vi "CMN_testmessage.vi"(8 "error in (no error)":errorcluster, 11 "message  in":string) -> (0 "error out":errorcluster, 1 "TIMEOUT":bool, 2 "ERROR":bool, 3 "message out":string)   [LabVIEW 2016]
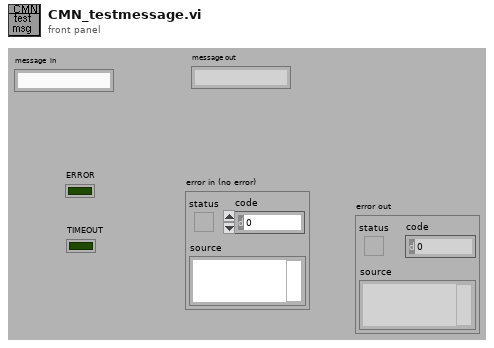
[diagram p1: front panel]
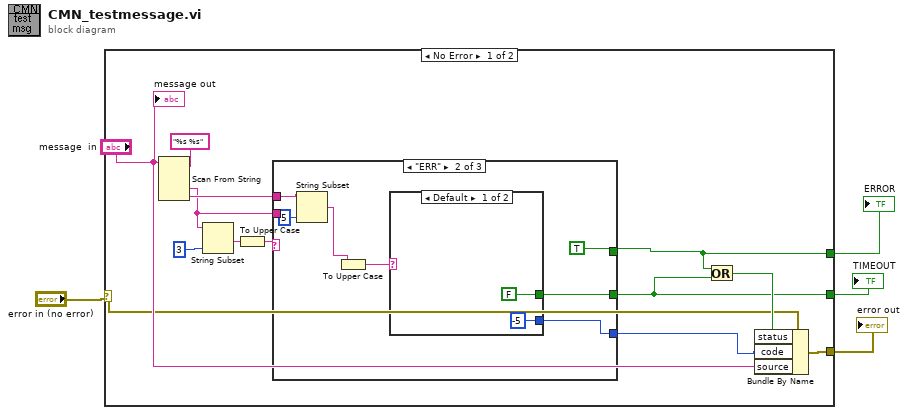
[diagram p0: block diagram]
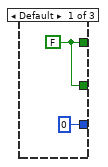
[diagram p2: hidden frame]
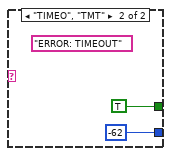
[diagram p3: hidden frame]
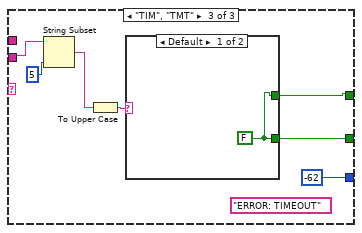
[diagram p4: hidden frame]
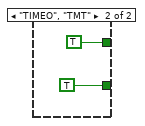
[diagram p5: hidden frame]
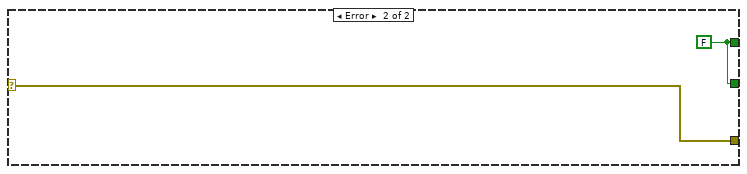
[diagram p6: hidden frame]
diagram:
  n1 = case shown="No Error" "error in (no error)" {
    selector: "error in (no error)" -> [w7 w41]
    tunnel: [w10 w41] -> w4
    tunnel: [w6 w42] -> w2
    tunnel: [w5 w42] -> w1
    frame No Error {
      n2 = Scan From String(format string="%s %s", input string="message  in") -> (output 1=w12:string, output 2=w13:string)  [unwired: 2 in, 5 out]
      n3 = String Subset(string=w12, length (rest)=3 ("length (rest)")) -> (substring=w15:string)  [unwired: 1 out]
      n4 = To Upper Case(1:w15) -> (0:w14:string)
      n5 = case shown="\"ERR\"" w14 {
        tunnel: [w19 TRUE w32] -> w5
        tunnel: w13 -> [_ w25 _]
        tunnel: [w19 w21 w34] -> w6
        tunnel: w12 -> [_ _ w33]
        tunnel: [0 w20 -62] -> w9
        frame Default {
          w19 = FALSE
        }
        frame "ERR" {
          n6 = String Subset(string=w25, length (rest)=5 ("length (rest)")) -> (substring=w23:string)  [unwired: 1 out]
          n7 = To Upper Case(1:w23) -> (0:w22:string)
          n8 = case shown="Default" w22 {
            tunnel: [FALSE TRUE] -> w21
            tunnel: [-5 -62] -> w20
            frame Default {
            }
            frame "TIMEO", "TMT" {
              (unwired) "ERROR: TIMEOUT"
            }
          }
        }
        frame "TIM", "TMT" {
          (unwired) "ERROR: TIMEOUT"
          n9 = String Subset(string=w33, length (rest)=5 ("length (rest)")) -> (substring=w36:string)  [unwired: 1 out]
          n10 = To Upper Case(1:w36) -> (0:w35:string)
          n11 = case shown="Default" w35 {
            tunnel: [w38 TRUE] -> w34
            tunnel: [w38 TRUE] -> w32
            frame Default {
              w38 = FALSE
            }
            frame "TIMEO", "TMT" {
            }
          }
        }
      }
      n12 = Or(x=w5, y=w6) -> (x .or. y?=w11:bool)
      n13 = Bundle By Name(cluster=w7, "status"=w11, "code"=w9, "source"="message  in") -> (w10:errorcluster)
      "message out" <- "message  in"
    }
    frame Error {
      w42 = FALSE
    }
  }
  "error out" <- w4
  "ERROR" <- w1
  "TIMEOUT" <- w2
